vi "ICM Main Path.vi"(8 "error in (no error)":errorcluster) -> (0 "error out":errorcluster, 2 "ICM Source Directory":path, 3 "ICM Root Path":path)   [LabVIEW 2024]
doc: "ICM Main Path.vi\n\nThis VI identifies the root path of the ICM system.\n\nInstrument Communication Module Version 1.0\nJuly, 2017 Original Code Consulting David Thomson\n www.originalcode.com"
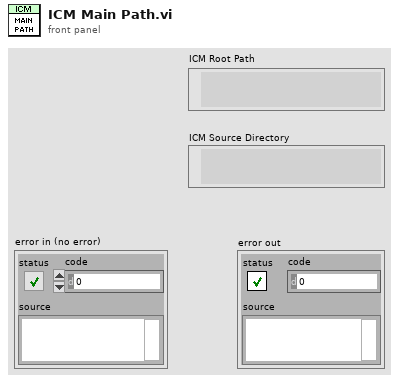
[diagram p1: front panel]
types:
  T1 = enum32{"invalid app kind", "Development System", "Run Time System", "Student Edition", "Embedded LabVIEW", "Evaluation", "Custom"}
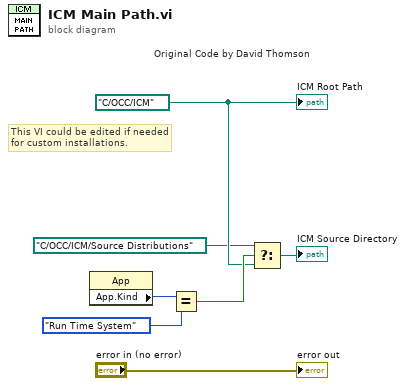
[diagram p0: block diagram]
diagram:
  w2 = path "C:/OCC/ICM"  # Original Code by David Thomson
  # "This VI could be edited if needed \nfor custom installations."
  n1 = property class="App"() -> ("App.Kind"=w6:T1)  [unwired: 2 in, 2 out]
  n2 = Equal?(x=w6, y=T1."Run Time System" ("Application:Kind")) -> (x = y?=w4:bool)
  n3 = Select(t=path "C:/OCC/ICM/Source Distributions", s=w4, f=w2) -> (s? t:f=→"ICM Source Directory":path)
  "ICM Root Path" <- w2
  "error out" <- "error in (no error)"
